vi "NI VeriStand - Get Timing and Sync Custom Device Is RTSI 0 Capable Flag.vi"(8 "error in (no error)":errorcluster, 11 "Device Ref in":T1 format="%.0x") -> (0 "error out":errorcluster, 2 "Is RTSI 0 Capable":bool, 3 "Device Ref out":T1 format="%.0x")   [LabVIEW 2020, in "Custom Device API.lvlib"]
doc: "Indicates whether the timing and sync custom device specified by <B>Device Ref in</B> can drive the RTSI 0 line. This line is a digital line that sends a clock signal that synchronizes all hardware I/O devices in the system."
uses:
  <vilib>/NI VeriStand/Custom Device API/Custom Device API.lvlib
  <vilib>/NI VeriStand/Custom Device API/Custom Device Item Ref.ctl
  <vilib>/NI VeriStand/Custom Device API/Get Item Property (Boolean).vi
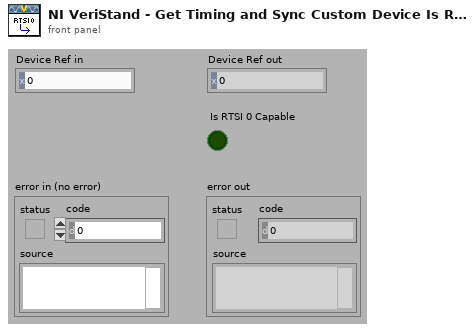
[diagram p1: front panel]
types:
  T1 = typedef "Custom Device API.lvlib/Custom Device Item Ref.ctl" = u64
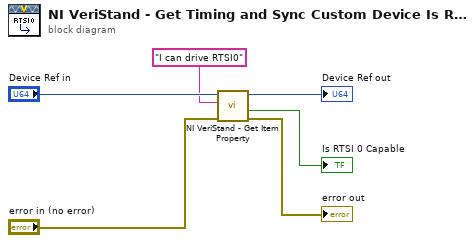
[diagram p0: block diagram]
diagram:
  n1 = call-poly <vilib>:"NI VeriStand - Get Item Property.vi"("error in (no error)"="error in (no error)", "Property Name"="I can drive RTSI0", "Item Ref in"="Device Ref in") -> ("error out"=→"error out":errorcluster, "Value"=→"Is RTSI 0 Capable":bool, "Item Ref out"=→"Device Ref out":T1)  [unwired: 1 in, 5 out]
